vi "Start Logging.vi"(8 "error in (no error)":errorcluster, 11 "Optimiser Cell in":refnum<class "Optimiser Cell.lvclass">) -> (0 "error out":errorcluster, 3 "Optimiser Cell out":refnum<class "Optimiser Cell.lvclass">)   [LabVIEW 2020, in "Run Utilities.lvlib" / "Optimiser Cell.lvclass"]
uses:
  Optimiser Cell.lvclass
  C:/Users/marco/Documents/GitHub_Lab/TALOS/talos/Run Utilities/Cell/Schedule Cell.lvclass
  Ancestor/Ancestor/Ancestor.lvclass/Ancestor.ctl
  Classes/Log/Log.lvclass/Log.ctl
  Optimiser Cell.lvclass/Optimiser Cell.ctl
  Support VIs/Generate Error.vi
  Classes/Log/Write.vi
  FGV/Error Memory/Get Error Description.vi
  Support VIs/Get PC name.vi
  Ancestor/Ancestor/Read ID.vi
  Support VIs/Get Class Name.vi
  <vilib>/Utility/error.llb/Clear Errors.vi
  FGV/Error Memory/Error Memory Core.vi
  <vilib>/AdvancedString/Delimited String to 1D String Array.vi
  Support VIs/Circus Root Path.vi
  FGV/Error Memory/Error Crt Lvl checker.vi
  FGV/Error Memory/Error Memory Core.vi/40c8088d-b597-4017-91af-faa98e00292e.vi
  FGV/Error Memory/Error Memory Core.vi/d4a3ab98-063c-4e44-b43d-fbdcfe6c2be2.vi
  Support VIs/Global Memory.vi
  <vilib>/Utility/LVClass/Get LV Class Name.vi
  Support VIs/Is in Packed Library.vi
  Support VIs/TALOS Root path.vi
  Support VIs/Read CSV worksheet.vi
  Support VIs/Global Constants.vi
  <vilib>/Utility/error.llb/General Error Handler.vi
  <vilib>/Utility/config.llb/Open Config Data.vi
  <vilib>/Utility/config.llb/Get Section Names.vi
  <vilib>/Utility/config.llb/Get Key Names.vi
  <vilib>/Utility/config.llb/Read Key.vi
  <vilib>/Utility/config.llb/Read Key (String).vi
  <vilib>/Utility/config.llb/Close Config Data.vi
  <vilib>/Utility/error.llb/Search and Replace Pattern.vi
  Classes/Log/Rotate.vi
  Support VIs/Error Log.vi
  Ancestor/Ancestor/Ancestor.lvclass
  <vilib>/Comparison/Equal/Equal Functor/Equal Functor.lvclass
  TALOS.lvlib
  Classes/Log/Log.lvclass
  C:/Users/marco/Documents/GitHub_Lab/TALOS/talos/Run Utilities/Optimiser Cell/Optimiser Cell.lvclass
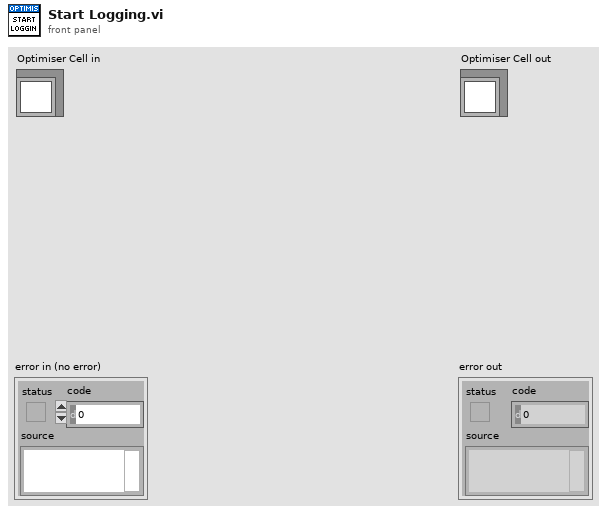
[diagram p1: front panel]
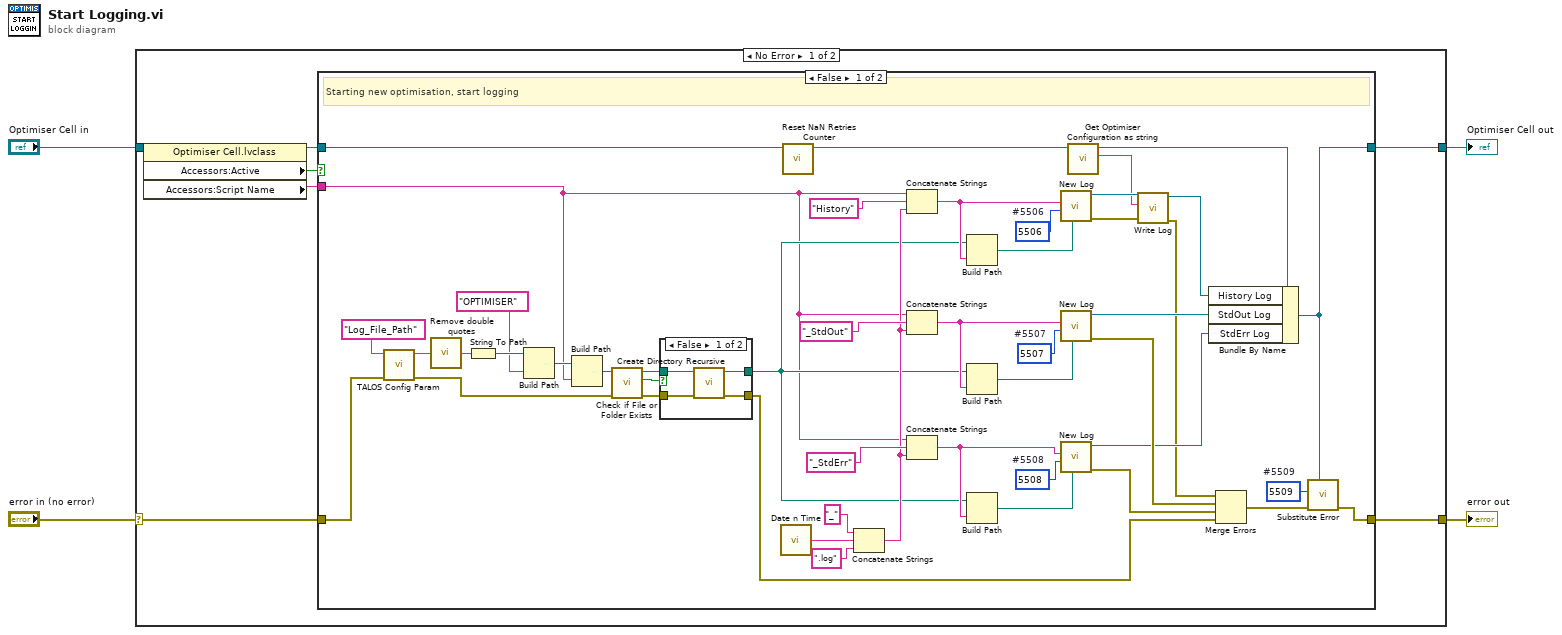
[diagram p0: block diagram]
diagram:
  n1 = case shown="No Error" "error in (no error)" {
    selector: "error in (no error)" -> [w9 w68]
    tunnel: [w10 w68] -> w3
    tunnel: [w11 w67] -> w1
    tunnel: "Optimiser Cell in" -> [w8 w67]
    frame No Error {
      n2 = property class="Optimiser Cell.lvclass"(reference=w8) -> (reference out=w7:refnum<class "Optimiser Cell.lvclass">, "Accessors:Active"=w5:bool, "Accessors:Script Name"=w6:string)  [unwired: 1 in, 1 out]
      n3 = case shown="False" w5 {
        tunnel: [w54 w66] -> w11
        tunnel: [w53 w65] -> w10
        tunnel: w9 -> [w47 w65]
        tunnel: w7 -> [w13 w66]
        tunnel: w6 -> [w14 _]
        frame False {
          w22 = 5509  # #5509
          w49 = 5508  # #5508
          w50 = 5507  # #5507
          w51 = 5506  # #5506
          # "Starting new optimisation, start logging"
          n4 = call "TALOS Config Param.vi"("error in (no error)"=w47, "Parameter Name"="Log_File_Path") -> ("error out"=w27:errorcluster, "Output"=w46:string)  [unwired: 8 in]
          n5 = call "Remove double quotes.vi"("Input string"=w46) -> ("Output string"=w45:string)  [unwired: 4 in]
          n6 = String To Path(string=w45) -> (path=w44:path)
          n7 = Build Path(base path=w44, name or relative path="OPTIMISER" ("Parameter Name")) -> (appended path=w42:path)
          n8 = Build Path(base path=w42, name or relative path=w14) -> (appended path=w28:path)
          n9 = call <vilib>:"Check if File or Folder Exists.vi"("error in (no error)"=w27, "path"=w28) -> ("error out"=w24:errorcluster, "file or folder exists?"=w26:bool, "dup path"=w25:path)  [unwired: 7 in]
          n10 = case shown="False" w26 {
            tunnel: w25 -> [w62 w64]
            tunnel: w24 -> [w61 w63]
            tunnel: [w60 w63] -> w21
            tunnel: [w59 w64] -> w23
            frame False {
              n11 = call <vilib>:"Create Directory Recursive.vi"("error in (no error)"=w61, "directory"=w62) -> ("error out"=w60:errorcluster, "directory copy"=w59:path)  [unwired: 3 in, 1 out]
            }
            frame True {
            }
          }
          n12 = call "Date n Time.vi"() -> ("Date & Time"=w40:string)  [unwired: 5 in]
          n13 = call-dynamic "Reset NaN Retries Counter.vi"("Run Optimiser in"=w13) -> ("Run Optimiser out"=w12:refnum<class "Optimiser Cell.lvclass">)  [unwired: 9 in, 1 out]
          n14 = Concatenate Strings("_" ("string"), w40, ".log" ("string")) -> (w32:string)
          n15 = Concatenate Strings(w14, "History" ("string"), w32) -> (w38:string)
          n16 = Concatenate Strings(w14, "_StdOut" ("string"), w32) -> (w37:string)
          n17 = Concatenate Strings(w14, "_StdErr" ("string"), w32) -> (w33:string)
          n18 = Build Path(base path=w23, name or relative path=w38) -> (appended path=w31:path)
          n19 = Build Path(base path=w23, name or relative path=w37) -> (appended path=w30:path)
          n20 = Build Path(base path=w23, name or relative path=w33) -> (appended path=w29:path)
          n21 = call "New Log.vi"("Path (optional)"=w31, "Specific Error Code"=w51, "Name"=w38) -> ("error out"=w18:errorcluster, "Log out"=w20:refnum<class "Log.lvclass">)  [unwired: 7 in]
          n22 = call "New Log.vi"("Path (optional)"=w30, "Specific Error Code"=w50, "Name"=w37) -> ("error out"=w58:errorcluster, "Log out"=w56:refnum<class "Log.lvclass">)  [unwired: 7 in]
          n23 = call "New Log.vi"("Path (optional)"=w29, "Specific Error Code"=w49, "Name"=w33) -> ("error out"=w57:errorcluster, "Log out"=w55:refnum<class "Log.lvclass">)  [unwired: 7 in]
          n24 = call-dynamic "Get Optimiser Configuration as string.vi"("Optimiser Cell in"=w12) -> ("Info"=w15:string, "Optimiser Cell out"=w16:refnum<class "Optimiser Cell.lvclass">)  [unwired: 8 in, 1 out]
          n25 = call "Write Log.vi"("error in (no error)"=w18, "Text"=w15, "Log in"=w20) -> ("error out"=w17:errorcluster, "Log out"=w19:refnum<class "Log.lvclass">)  [unwired: 7 in]
          n26 = Bundle By Name(cluster=w16, "History Log"=w19, "StdOut Log"=w56, "StdErr Log"=w55) -> (w54:refnum<class "Optimiser Cell.lvclass">)
          n27 = Merge Errors(w17, w58, w57, w21) -> (w52:errorcluster)
          n28 = call "Substitute Error.vi"("LabVIEW Object"=w54, "error in (no error)"=w52, "Error Code"=w22) -> ("error out"=w53:errorcluster)  [unwired: 8 in]
        }
        frame True {
          # "Logs already created, do nothing"
        }
      }
    }
    frame Error {
    }
  }
  "error out" <- w3
  "Optimiser Cell out" <- w1
